vi "write_params.vi"(8 "error in (no error)":errorcluster, 10 "params":T1={"estimators"=[], "cv"=5.0, "n_jobs"=1.0, "passthrough"=FALSE, "verbose"=0.0}, 11 "StackingRegressor in":refnum<class "StackingRegressor.lvclass">) -> (0 "error out":errorcluster, 3 "StackingRegressor out":refnum<class "StackingRegressor.lvclass">)   [LabVIEW 2020, in "StackingRegressor.lvclass"]
uses:
  StackingRegressor.lvclass
  Controls/stacking_regressor_params.ctl
  StackingRegressor.lvclass/StackingRegressor.ctl
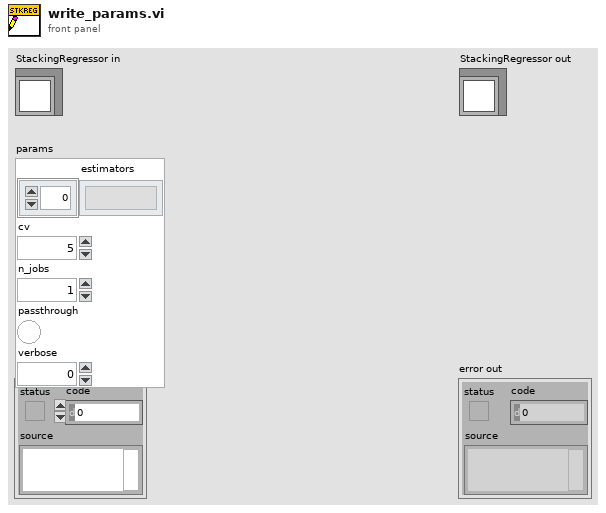
[diagram p1: front panel]
types:
  T1 = typedef "stacking_regressor_params.ctl" = cluster{"estimators":string[], "cv":dbl, "n_jobs":dbl, "passthrough":bool, "verbose":dbl}
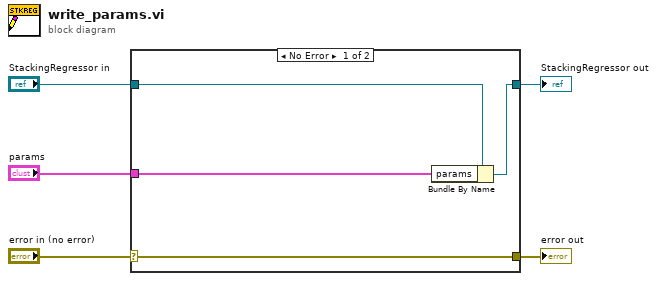
[diagram p0: block diagram]
diagram:
  n1 = case shown="No Error" "error in (no error)" {
    selector: "error in (no error)" -> [w9 w10]
    tunnel: [w9 w10] -> w4
    tunnel: [w7 w11] -> w2
    tunnel: "StackingRegressor in" -> [w8 w11]
    tunnel: "params" -> [w6 _]
    frame No Error {
      n2 = Bundle By Name(cluster=w8, "params"=w6) -> (w7:refnum<class "StackingRegressor.lvclass">)
    }
    frame Error {
    }
  }
  "error out" <- w4
  "StackingRegressor out" <- w2
